vi "Sample Transfer go for State.vi"(4 "Publish? (T)":bool=TRUE, 5 "Milliseconds To Wait (1000)":i32=1000, 6 "Really? (T)":bool=TRUE, 7 "Restart Message (F)":bool, 8 "error in (no error)":errorcluster, 9 "State Timeout (Inf=no timeout )":dbl=inf, 10 "Sample Transfer State":T1, 11 "cRIO-CO2 in":refnum<class "cRIO-CO2.lvclass">) -> (0 "error out":errorcluster, 3 "cRIO-CO2 out":refnum<class "cRIO-CO2.lvclass">)   [LabVIEW 2015, in "cRIO-Carbondioxide.lvlib" / "cRIO-CO2.lvlib" / "cRIO-CO2.lvclass"]
uses:
  cRIO-CO2.lvclass
  Controls/Sample Transfer State Enumerator.ctl
  cRIO-CO2.lvclass/cRIO-CO2.ctl
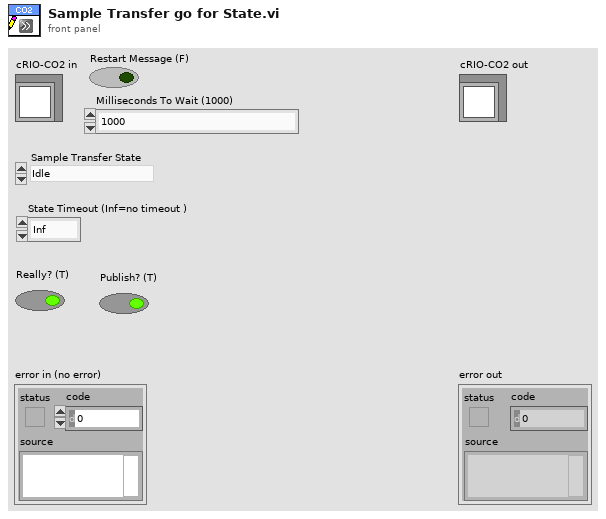
[diagram p1: front panel]
types:
  T1 = typedef "Sample Transfer State Enumerator.ctl" = enum16{"Idle", "Initialize", "Check Containers", "Check Temperatures", "Start Turbo", "Warm Up Containers", "Prepare for purging", "Purge Capillary", "Purge", "Open Containers", "Introduce Sample", "Measure Base Pressure", "Home Syringe", "Start Freezer", "Freeze Target", "Crystalize", "Initiate Stash", "Stash", "Polish", "Stop Freezers", "Push Sample", "Complete", "Abort", "Error", "Undefined"}
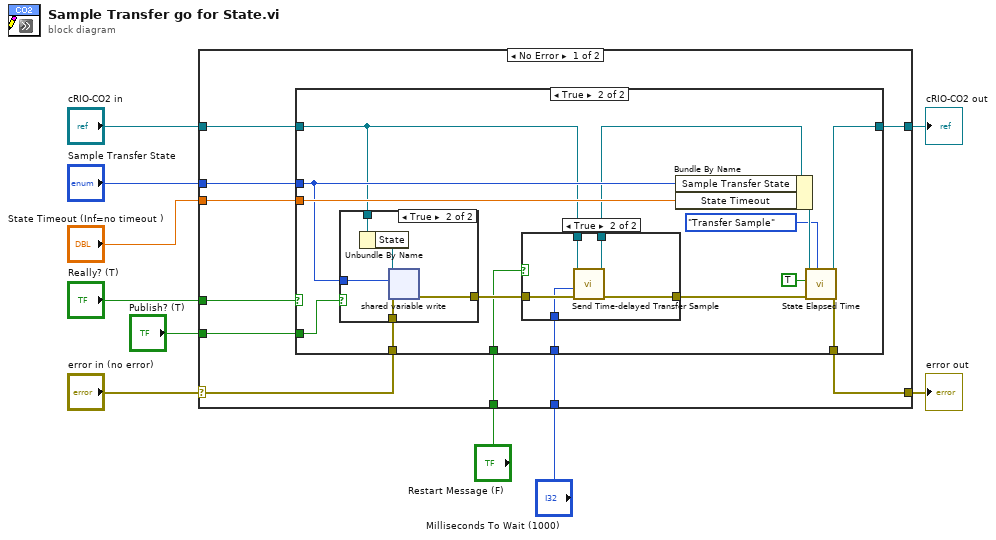
[diagram p0: block diagram]
diagram:
  n1 = case shown="No Error" "error in (no error)" {
    selector: "error in (no error)" -> [w20 w51]
    tunnel: [w17 w51] -> w9
    tunnel: [w13 w52] -> w7
    tunnel: "cRIO-CO2 in" -> [w14 w52]
    tunnel: "Sample Transfer State" -> [w19 _]
    tunnel: "State Timeout (Inf=no timeout )" -> [w18 _]
    tunnel: "Really? (T)" -> [w16 _]
    tunnel: "Publish? (T)" -> [w15 _]
    tunnel: "Restart Message (F)" -> [w12 _]
    tunnel: "Milliseconds To Wait (1000)" -> [w11 _]
    frame No Error {
      n2 = case shown="True" w16 {
        tunnel: w20 -> [w22 w37]
        tunnel: w19 -> [_ w31]
        tunnel: w18 -> [_ w36]
        tunnel: [w22 w35] -> w17
        tunnel: w15 -> [_ w30]
        tunnel: w14 -> [w21 w26]
        tunnel: [w21 w29] -> w13
        tunnel: w12 -> [_ w24]
        tunnel: w11 -> [_ w23]
        frame False {
        }
        frame True {
          n3 = case shown="True" w30 {
            tunnel: w37 -> [w45 w47]
            tunnel: [w45 w49] -> w28
            tunnel: w31 -> [_ w48]
            tunnel: w26 -> [_ w50]
            frame False {
            }
            frame True {
              n4 = Unbundle By Name(w50) -> ("State"=w46:refnum<k21>)
              n5 = shared-variable-write(w46, w47, w48) -> (w49:errorcluster)  [unwired: 1 out]
            }
          }
          n6 = case shown="True" w24 {
            tunnel: w28 -> [w39 w44]
            tunnel: [w39 w43] -> w27
            tunnel: w26 -> [w38 w42]
            tunnel: [w38 w41] -> w25
            tunnel: w23 -> [_ w40]
            frame False {
            }
            frame True {
              n7 = call "Send Time-delayed Transfer Sample.vi"("error in (no error)"=w44, "Milliseconds To Wait (1000)"=w40, "cRIO-CO2 in"=w42) -> ("error out"=w43:errorcluster, "cRIO-CO2 out"=w41:refnum<class "cRIO-CO2.lvclass">)  [unwired: 7 in]
            }
          }
          n8 = Bundle By Name(cluster=w25, "Sample Transfer State"=w31, "State Timeout"=w36) -> (w34:refnum<class "cRIO-CO2.lvclass">)
          n9 = call "State Elapsed Time.vi"("State Machine"=enum16{"Transfer Sample", "Push Sample"}."Transfer Sample", "error in (no error)"=w27, "Reset (F)"=TRUE, "cRIO-CO2 in"=w34) -> ("error out"=w35:errorcluster, "cRIO-CO2 out"=w29:refnum<class "cRIO-CO2.lvclass">)  [unwired: 4 in, 2 out]
        }
      }
    }
    frame Error {
    }
  }
  "error out" <- w9
  "cRIO-CO2 out" <- w7
